vi "forceOutputState.vi"(8 "error in (no error)":errorcluster, 9 "data":T1(array[cluster]), 10 "physicalChannels":string[](array[string]), 11 "k3390_AWG in":refnum<class "k3390_AWG.lvclass">) -> (0 "error out":errorcluster, 3 "k3390_AWG out":refnum<class "k3390_AWG.lvclass">)   [LabVIEW 2009, in "Hardware.lvlib" / "Channels.lvlib" / "k3390_AWG.lvclass"]
uses:
  k3390_AWG.lvclass
  k3390_AWG.lvclass/k3390_AWG.ctl
  <instrlib>/Keithley 3390/Public/Configure/Configure Waveform (Sine).vi
  <instrlib>/Keithley 3390/Keithley 3390.lvlib
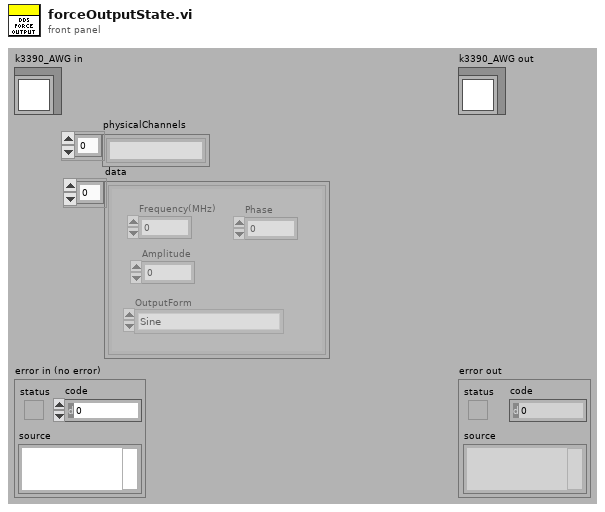
[diagram p1: front panel]
types:
  T1 = cluster{"Frequency(MHz)":dbl, "Amplitude":dbl, "Phase":dbl, "OutputForm":enum16{"Sine", "Square", "Triangle", "Arbitrary"}}[]
  T2 = cluster{"Frequency(MHz)":dbl, "Amplitude":dbl, "Phase":dbl, "OutputForm":enum16{"Sine", "Square", "Triangle", "Arbitrary"}}
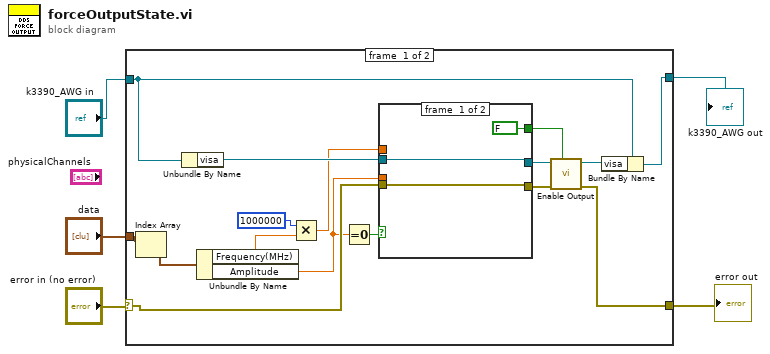
[diagram p0: block diagram]
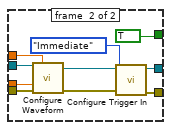
[diagram p2: hidden frame]
diagram:
  n1 = case shown="No Error" "error in (no error)" {
    selector: "error in (no error)" -> [w17 w35]
    tunnel: "k3390_AWG in" -> [w20 w36]
    tunnel: [w19 w36] -> w3
    tunnel: [w18 w35] -> w2
    tunnel: "data" -> [w21 _]
    frame #0 {
      n2 = Index Array(array=w21) -> (element=w16:T2)  [unwired: 1 in]
      n3 = Unbundle By Name(w20) -> ("visa"=w15:refnum<visa-resource-name>)
      n4 = Unbundle By Name(w16) -> ("Frequency(MHz)"=w9:dbl, "Amplitude"=w6:dbl)
      n5 = Multiply(x=1000000, y=w9) -> (x*y=w8:dbl)
      n6 = Equal To 0?(x=w6) -> (x = 0?=w7:bool)
      n7 = case shown="False" w7 {
        tunnel: w15 -> [w24 w34]
        tunnel: w8 -> [_ w33]
        tunnel: w6 -> [_ w32]
        tunnel: [w24 w28] -> w14
        tunnel: [w23 w27] -> w13
        tunnel: w17 -> [w23 w26]
        tunnel: [FALSE TRUE] -> w11
        frame #0 {
        }
        frame #1 {
          n8 = call-poly <instrlib>:"Configure Waveform.vi"("VISA resource name"=w34, "Frequency (1000 Hz)"=w33, "Amplitude (1.0 Vpp)"=w32, "error in (no error)"=w26) -> ("VISA resource name out"=w31:refnum<visa-resource-name>, "error out"=w30:errorcluster)  [unwired: 10 in]
          n9 = call <instrlib>:"Configure Trigger In.vi"("error in (no error)"=w30, "Trigger Source (0:Immediate)"=enum16{"Immediate", "External", "Bus"}."Immediate", "VISA resource name"=w31) -> ("error out"=w27:errorcluster, "VISA resource name out"=w28:refnum<visa-resource-name>)  [unwired: 7 in]
        }
      }
      n10 = call <instrlib>:"Enable Output.vi"("Enable Output (T: Enable)"=w11, "error in (no error)"=w13, "VISA resource name"=w14) -> ("error out"=w18:errorcluster, "VISA resource name out"=w12:refnum<visa-resource-name>)  [unwired: 7 in]
      n11 = Bundle By Name(cluster=w20, "visa"=w12) -> (w19:refnum<class "k3390_AWG.lvclass">)
    }
    frame #1 {
    }
  }
  "error out" <- w2
  "k3390_AWG out" <- w3
